vi "FMS Data Array.vi"   [LabVIEW 2017]
uses:
  <vilib>/Rock Robotics/Network Tables/NT Write String Array.vi
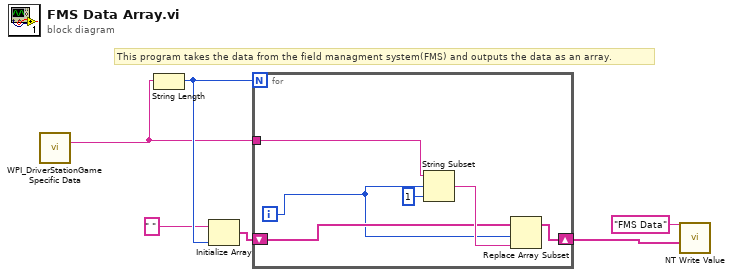
[diagram p0: block diagram]
diagram:
  # "This program takes the data from the field managment system(FMS) and outputs the data as an array."
  n1 = call <vilib>:"WPI_DriverStationGame Specific Data.vi"() -> ("Game Specific Data"=w1:string)  [unwired: 11 in]
  n2 = String Length(string=w1) -> (length=w6:i32)
  n3 = Initialize Array(" ", w6) -> (w4:string[])
  n4 = for {
    N: w6 -> [_]
    shift-right: [w9] -> w3
    shift-left: w4 -> [w10]
    tunnel: w1 -> [w7]
    i -> [w8]
    n5 = String Subset(string=w7, offset (0)=w8, length (rest)=1 ("length (rest)")) -> (substring=w11:string)
    n6 = Replace Array Subset(array=w10, new element=w11, index=w8) -> (w9:string[])
  }
  n7 = call-poly <vilib>:"NT Write Value.vi"("String Array"=w3, "Name"="FMS Data") -> ()  [unwired: 9 in, 1 out]
